vi "Set_Measurement_Conditions.vi"(3 "Simulate/Run":T3, 4 "Currently on Point":i32=11, 5 "Traverse line":T5 {"Carrier_2 Q (l/min)" format="%#.2f"; "Row Duration (mins)" format="%#.1f"; "Row No" min=0; "Trace Gas Concentration (%)" min=0.0 format="%#_4f"; "Carrier_1 Q (l/min)" format="%#.2f"; "Tunnel Speed" format="%#.2f"; "Start X" format="%#.2f"; "Start Y" format="%#.2f"; "Start Z" format="%#.2f"; "End X" format="%#.2f"; "End Y" format="%#.2f"; "End Z" format="%#.2f"; "Averaging time (min)" min=0.0 format="%#.2f"}) -> (0 "Status Cluster":T1)   [LabVIEW 2016]
uses:
  Traverse_cluster.ctl
  Spacing.ctl
  Controls/Multi_run_mode.ctl
  Execute_case.ctl
  Controls/User_Specific_mode.ctl
  Status_Cluster.ctl
  Multi_Run_Status.ctl
  ADAM Client/Sub VIs/ADAM Controls/Client_Source_Status.ctl
  Globals/Preference_global.vi
  Globals/Extra_Commands_Global.vi
panel:
  out "Heaters On?":bool
  out "Time Source Started":dbl
  out "Execute Case":T4=enum."Set All Conditions"
  # "X           Y            Z"
  # "Start"
  # "End"
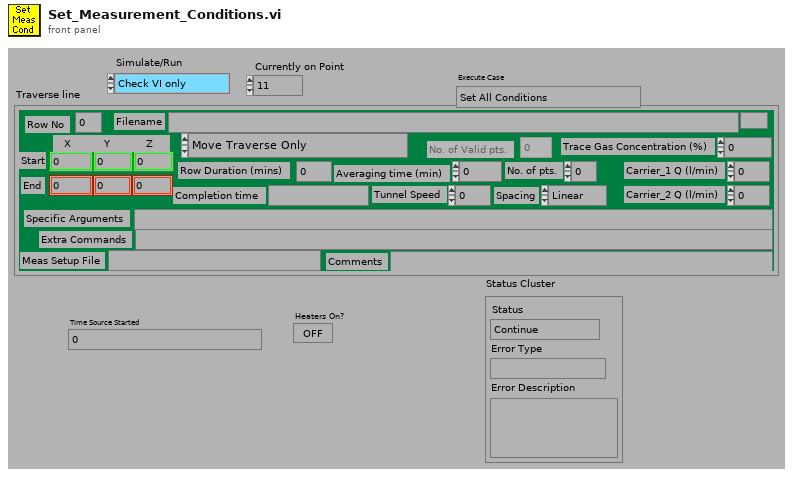
[diagram p1: front panel]
types:
  T1 = typedef "Status_Cluster.ctl" = cluster{"Status":T2, "Error Type":string, "Error Description":string}
  T2 = typedef "Multi_Run_Status.ctl" = enum16{"Continue", "Continue with Error", "Jump to Next Point", "Jump to Next Row", "Jump To Fall Back", "Terminate Run"}
  T3 = typedef "User_Specific_mode.ctl" = enum16{"Check VI only", "Run VI"}
  T4 = typedef "Execute_case.ctl" = enum16{"Start", "EnFlo Tunnel Check", "Set All Conditions", "Establish Exp Conditions", "The End"}
  T5 = typedef "Traverse_cluster.ctl" = cluster{"Start X":sgl, "Start Y":sgl, "Start Z":sgl, "End X":sgl, "End Y":sgl, "End Z":sgl, "No. of pts.":i32, "Spacing":T6, "Filename":path, "Tunnel Speed":dbl, "Averaging time (min)":dbl, "Extra Commands":string, "Carrier_1 Q (l/min)":dbl, "Carrier_2 Q (l/min)":dbl, "Trace Gas Concentration (%)":dbl, "Specific Arguments":string, "Comments":string, "Row No":i32, "Row Type Selector":T7, "Completion time":string, "Row Duration (mins)":dbl, "No. of Valid pts.":i32, "Meas Setup File":string}
  T6 = typedef "Spacing.ctl" = enum16{"Linear", "Log", "Gauss", "Specified", "N/A"}
  T7 = typedef "Multi_run_mode.ctl" = enum16{"Move Traverse Only", "Set Tunnel Speed Only", "Set Source Only", "Set Measurement Conditions", "Single Measurement", "Vertical Profile", "Lateral Profile", "Longitudinal Profile", "Explore Volume", "Multi-Axis Profile", "Auto Calibrate", "Meas Fast FID Bkgnd", "Check Beam Power", "Scanning Valve Measurement", "Run VI Named:", "Set ADAM Ch", "Wait (minutes)", "Send Message", "Synchronize With:", "Fall Back to this Row", "Turn Off Row Repeating", "Blank Row", "Traverse 3D Volume"}
  T8 = typedef "Client_Source_Status.ctl" = enum16{"Not Using", "Using", "Must Have"}
  T9 = typedef "Server_Comms.ctl" = enum16{"Server Link Healthy", "Do Not Link To Server"}
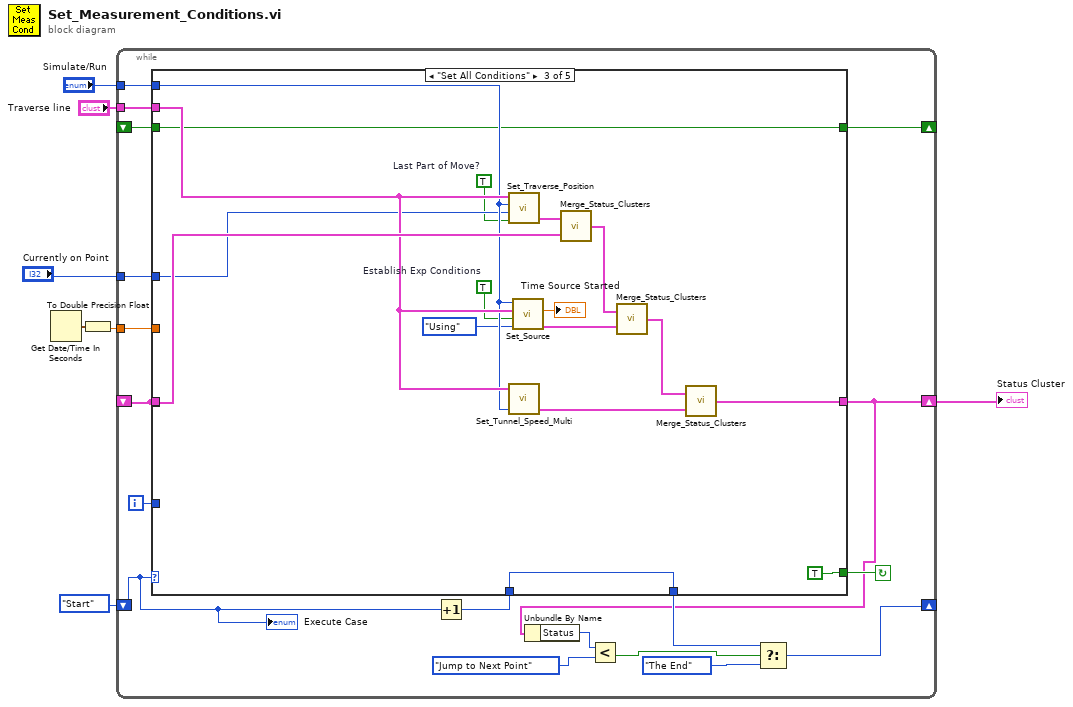
[diagram p0: block diagram]
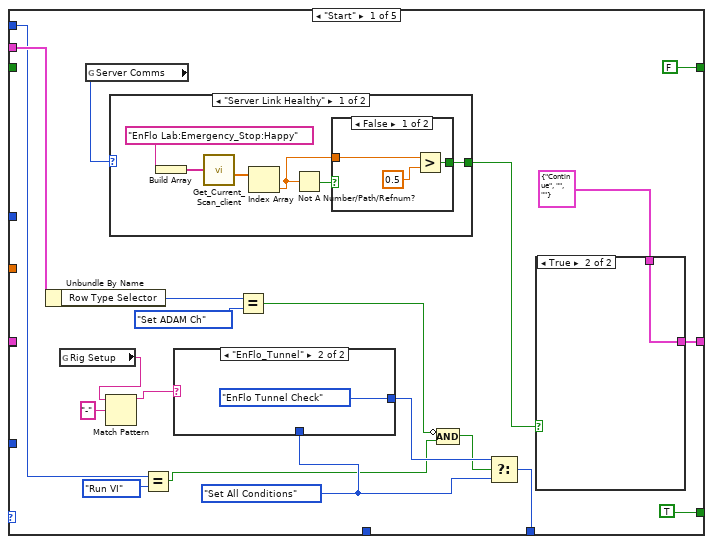
[diagram p2: hidden frame]
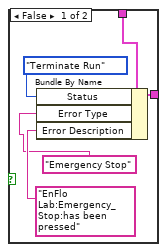
[diagram p3: hidden frame]
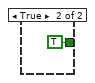
[diagram p4: hidden frame]
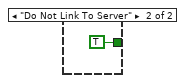
[diagram p5: hidden frame]
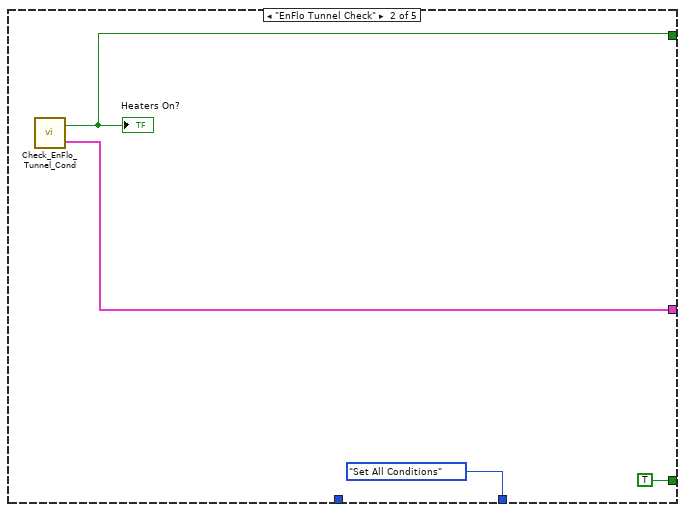
[diagram p7: hidden frame]
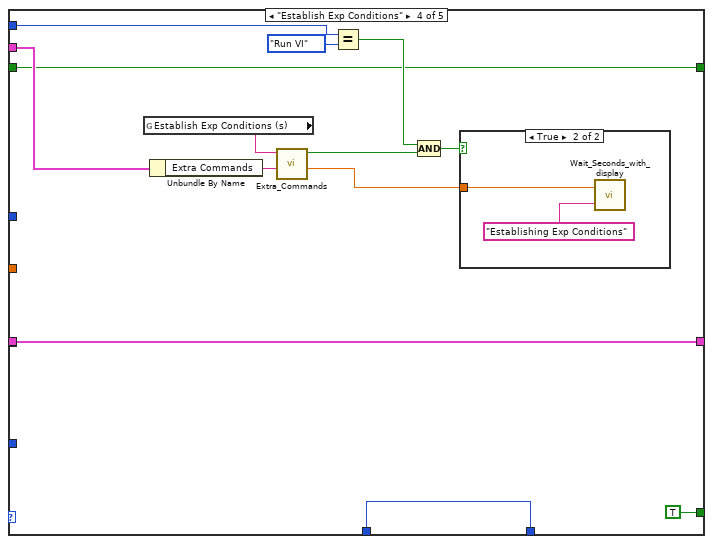
[diagram p8: hidden frame]
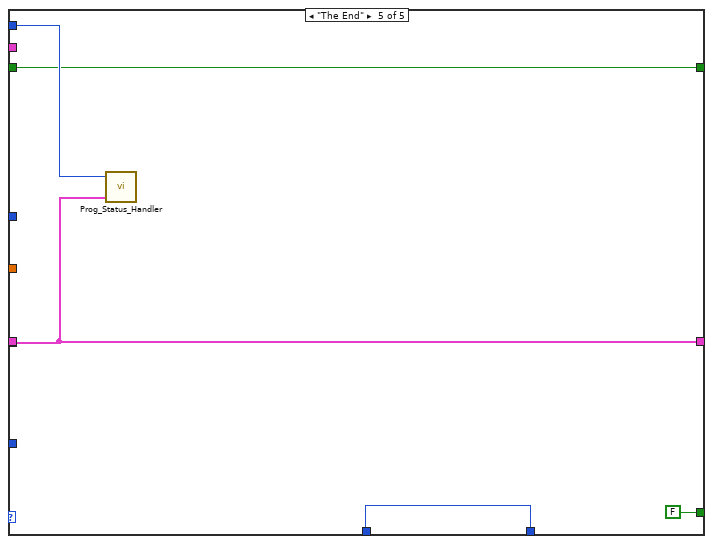
[diagram p10: hidden frame]
diagram:
  n1 = Get Date/Time In Seconds() -> (seconds since 1Jan1904=w1:timestamp)
  n2 = To Double Precision Float(number=w1) -> (double precision float=w2:dbl)
  n3 = while {
    tunnel: w2 -> [w15]
    tunnel: "Traverse line" -> [w16]
    tunnel: "Currently on Point" -> [w17]
    shift-left: _ -> [w18]
    shift-right: [w11] -> w4
    tunnel: "Simulate/Run" -> [w22]
    shift-left: Execute_case."Start" ("Execute Case") -> [w23]
    shift-right: [w20] -> _
    shift-right: [w13] -> _
    shift-left: _ -> [w12]
    i -> [w14]
    stop <- w25 continue-if-true
    n4 = Increment(x=w23) -> (x+1=w24:T4)
    n5 = case shown="\"Set All Conditions\"" w23 {
      tunnel: [TRUE TRUE TRUE TRUE FALSE] -> w25
      tunnel: w24 -> [_ _ w80 w89 w104]
      tunnel: w22 -> [w43 _ w78 w97 w103]
      tunnel: w18 -> [_ _ w84 w88 w101]
      tunnel: [w27 w65 w81 w88 w101] -> w11
      tunnel: [w40 Execute_case."Set All Conditions" ("Execute Case") w80 w89 w104] -> w19
      tunnel: w18 -> [_ _ _ _ _]
      tunnel: w17 -> [_ _ w77 _ _]
      tunnel: w16 -> [w45 _ w83 w96 _]
      tunnel: w15 -> [_ _ _ _ _]
      tunnel: w14 -> [_ _ _ _ _]
      tunnel: [FALSE w66 w74 w87 w102] -> w13
      tunnel: w12 -> [_ _ w74 w87 w102]
      frame "Start" {
        w41 = Execute_case."Set All Conditions" ("Execute Case")
        n6 = Unbundle By Name(w45) -> ("Row Type Selector"=w35:T7)
        n7 = global read "Preference_global.vi" "Rig Setup"() -> (w33:string)
        n8 = global read "Preference_global.vi" "Server Comms"() -> (w30:T9)
        n9 = Match Pattern(string=w33, regular expression="-") -> (before substring=w32:string)  [unwired: 4 out]
        n10 = case shown="\"Server Link Healthy\"" w30 {
          tunnel: [w52 TRUE] -> w29
          frame "Server Link Healthy" {
            n11 = Build Array("EnFlo Lab:Emergency_Stop:Happy") -> (w55:string[])
            n12 = call "Get_Current_Scan_client.vi"("ADAM Ch Names"=w55) -> ("Numerical Values"=w57:dbl[])  [unwired: 1 in, 2 out]
            n13 = Index Array(array=w57) -> (element=w53:dbl)  [unwired: 1 in]
            n14 = Not A Number/Path/Refnum?(number/path/refnum=w53) -> (NaN/Path/Refnum?=w54:bool)
            n15 = case shown="False" w54 {
              tunnel: w53 -> [w60 _]
              tunnel: [w58 TRUE] -> w52
              frame False {
                n16 = Greater?(x=w60, y=0.5) -> (0:w58:bool)
              }
              frame True {
              }
            }
          }
          frame "Do Not Link To Server" {
          }
        }
        n17 = Equal?(x=w43, y=User_Specific_mode."Run VI" ("Simulate/Run")) -> (x = y?=w37:bool)
        n18 = case shown="\"EnFlo_Tunnel\"" w32 {
          tunnel: [w63 Execute_case."EnFlo Tunnel Check" ("Execute Case")] -> w42
          tunnel: w41 -> [w63 _]
          frame "Other", Default {
          }
          frame "EnFlo_Tunnel" {
          }
        }
        n19 = Equal?(x=w35, y=Multi_run_mode."Set ADAM Ch" ("Mode")) -> (x = y?=w38:bool)
        n20 = Compound Arithmetic op=AND(invert w38, w37) -> (w36:bool)
        n21 = Select(t=w42, s=w36, f=w41) -> (s? t:f=w40:T4)
        n22 = case shown="True" w29 {
          tunnel: T1 {"Status"=enum."Continue", "Error Type"="", "Error Description"=""} ("Status Cluster") -> [w50 w51]
          tunnel: [w49 w51] -> w27
          frame False {
            n23 = Bundle By Name(cluster=w50, "Status"=Multi_Run_Status."Terminate Run", "Error Type"="Emergency Stop", "Error Description"="EnFlo Lab:Emergency_Stop:has been pressed") -> (w49:T1)
          }
          frame True {
          }
        }
      }
      frame "EnFlo Tunnel Check" {
        n24 = call "Check_EnFlo_Tunnel_Cond.vi"() -> ("Status Cluster"=w65:T1, "Heaters On?"=w66:bool)  [unwired: 2 in]
        "Heaters On?" <- w66
      }
      frame "Set All Conditions" {
        w69 = TRUE  # Last Part of Move?
        w70 = TRUE  # Establish Exp Conditions
        n25 = call "Set_Traverse_Position.vi"("Last Part of Move?"=w69, "Currently on Point"=w77, "Simulate/Run"=w78, "Traverse line"=w83) -> ("Status Cluster"=w71:T1)  [unwired: 2 in]
        n26 = call "Set_Tunnel_Speed_Multi.vi"("Simulate/Run"=w78, "Traverse line"=w83) -> ("Status Cluster"=w82:T1)  [unwired: 3 out]
        n27 = call "Set_Source.vi"("Source Status"=Client_Source_Status."Using", "Establish Exp Conditions"=w70, "Traverse line"=w83, "Simulate/Run"=w78) -> ("Status Cluster"=w72:T1, "Time Source Started"=→"Time Source Started":dbl)  [unwired: 4 out]
        n28 = call "Merge_Status_Clusters.vi"("Status Cluster 2"=w84, "Status Cluster 1"=w71) -> ("Status Cluster Out"=w76:T1)
        n29 = call "Merge_Status_Clusters.vi"("Status Cluster 2"=w72, "Status Cluster 1"=w76) -> ("Status Cluster Out"=w75:T1)
        n30 = call "Merge_Status_Clusters.vi"("Status Cluster 2"=w82, "Status Cluster 1"=w75) -> ("Status Cluster Out"=w81:T1)
      }
      frame "Establish Exp Conditions" {
        n31 = global read "Extra_Commands_Global.vi" "Establish Exp Conditions (s)"() -> (w95:string)
        n32 = Unbundle By Name(w96) -> ("Extra Commands"=w90:string)
        n33 = call "Extra_Commands.vi"("String to Search"=w90, "Command"=w95) -> ("Numeric Value"=w86:dbl, "Command Found"=w92:bool)  [unwired: 1 in, 3 out]
        n34 = Equal?(x=w97, y=User_Specific_mode."Run VI" ("Simulate/Run")) -> (x = y?=w91:bool)
        n35 = Compound Arithmetic op=AND(w91, w92) -> (w93:bool)
        n36 = case shown="True" w93 {
          tunnel: w86 -> [_ w99]
          frame False {
          }
          frame True {
            n37 = call "Wait_Seconds_with_display.vi"("Message"="Establishing Exp Conditions", "Seconds to wait"=w99) -> ()  [unwired: 2 out]
          }
        }
      }
      frame "The End" {
        n38 = call "Prog_Status_Handler.vi"("Status Cluster"=w101, "Simulate/Run"=w103) -> ()  [unwired: 2 out]
      }
    }
    n39 = Unbundle By Name(w11) -> ("Status"=w10:T2)
    n40 = Less?(x=w10, y=Multi_Run_Status."Jump to Next Point" ("Status")) -> (x < y?=w8:bool)
    n41 = Select(t=w19, s=w8, f=Execute_case."The End" ("Execute Case")) -> (s? t:f=w20:T4)
    "Execute Case" <- w23
  }
  "Status Cluster" <- w4
